vi "FTW-CodeGen-BuildMenu5.vi"(0 "State In":T2, 5 "XRef":refnum<vi>, 7 "MenuRef":refnum<k9>, 9 "Point":cluster{"H":i32, "V":i32}, 11 "Menu Type":T1(ring)) -> ()   [LabVIEW 2015, in "FTW-Dataflow-Burrow.xnode"]
uses:
  FTW-Dataflow-Burrow.xnode
  FTW-CodeGen-State.ctl
panel:
  # "Inputs"
  # "Outputs"
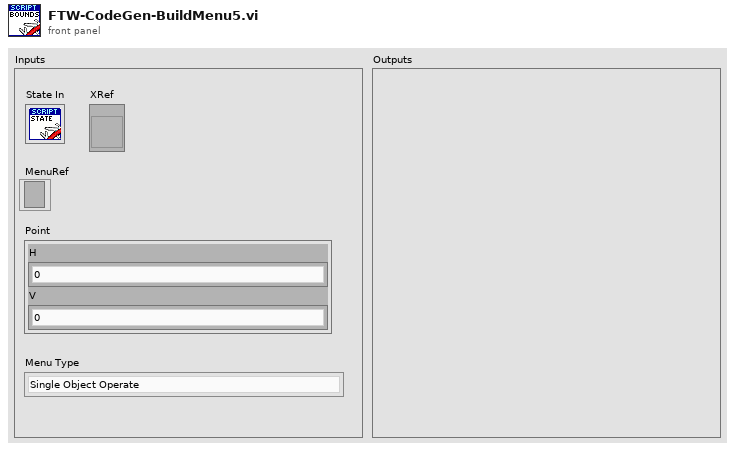
[diagram p1: front panel]
types:
  T1 = enum32{"Single Object Operate", "Single Object Popup", "Multi Object Popup Master", "Multi Object Popup Other"}
  T2 = typedef "FTW-Dataflow-Burrow.xnode/FTW-CodeGen-State.ctl" = cluster{"InputTerminals":cluster{"Wired?":bool, "ID":string, "DataName":string, "DataColor":u32, "Type":variant}[], "EnableTiming?":bool}
  T3 = cluster{"Wired?":bool, "ID":string, "DataName":string, "DataColor":u32, "Type":variant}[]
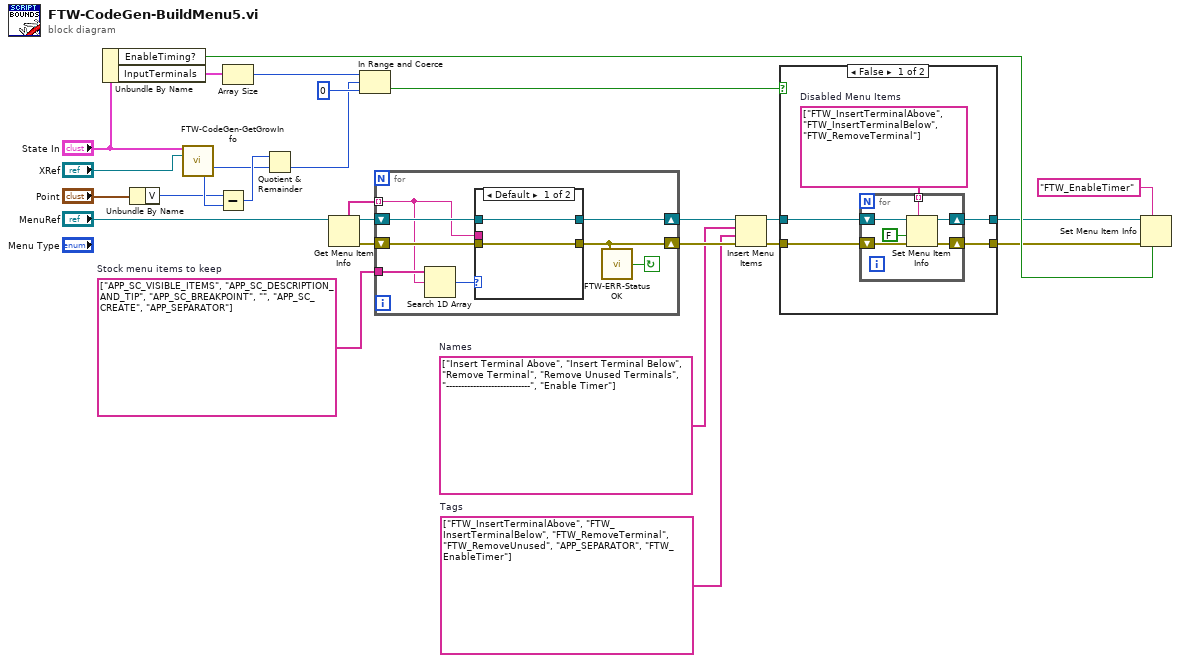
[diagram p0: block diagram]
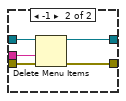
[diagram p3: hidden frame]
diagram:
  w19 = string[] ["FTW_InsertTerminalAbove", "FTW_InsertTerminalBelow", "FTW_RemoveTerminal", "FTW_RemoveUnused", "APP_SEPARATOR", "FTW_EnableTimer"]  # Tags
  w20 = string[] ["Insert Terminal Above", "Insert Terminal Below", "Remove Terminal", "Remove Unused Terminals", "----------------------------", "Enable Timer"]  # Names
  w25 = string[] ["APP_SC_VISIBLE_ITEMS", "APP_SC_DESCRIPTION_AND_TIP", "APP_SC_BREAKPOINT", "", "APP_SC_CREATE", "APP_SEPARATOR"]  # Stock menu items to keep
  n1 = Unbundle By Name("State In") -> ("EnableTiming?"=w17:bool, "InputTerminals"=w1:T3)
  n2 = Unbundle By Name("Point") -> ("V"=w13:i32)
  n3 = call "FTW-CodeGen-GetGrowInfo.vi"("State In"="State In", "XRef"="XRef") -> ("Terminal Height"=w14:i32, "Total Top Banner Height"=w16:i32)  [unwired: 5 in, 7 out]
  n4 = Subtract(x=w13, y=w16) -> (x-y=w15:i32)
  n5 = Array Size(array=w1) -> (size(s)=w8:i32)
  n6 = Quotient & Remainder(x=w15, y=w14) -> (floor(x/y)=w7:i32)  [unwired: 1 out]
  n7 = Get Menu Item Info(11:"MenuRef") -> (0:w23:errorcluster, 3:w26:refnum<k9>, 5:w24:string[])  [unwired: 2 in, 4 out]
  n8 = In Range and Coerce(upper limit=w8, x=w7, lower limit=0) -> (In Range?=w2:bool)  [unwired: 1 out]
  n9 = for {
    shift-right: [w35] -> w21
    shift-left: w26 -> [w34]
    tunnel: w25 -> [w33]
    tunnel: w24 -> [w30] mode=indexing
    shift-right: [w29] -> w22
    shift-left: w23 -> [w31]
    stop <- w28 continue-if-true
    n10 = Search 1D Array(1D array=w33, element=w30) -> (index of element=w32:i32)  [unwired: 1 in]
    n11 = case shown="Default" w32 {
      tunnel: [w37 w42] -> w35
      tunnel: w34 -> [w37 w41]
      tunnel: w31 -> [w36 w40]
      tunnel: [w36 w39] -> w29
      tunnel: w30 -> [_ w38]
      frame Default {
      }
      frame -1 {
        n12 = Delete Menu Items(6:w40, 7:w38, 9:w41) -> (0:w39:errorcluster, 3:w42:refnum<k9>)  [unwired: 1 in]
      }
    }
    n13 = call "FTW-ERR-StatusOK.vi"("error to check"=w29) -> ("Status OK?"=w28:bool)
  }
  n14 = Insert Menu Items(6:w22, 7:w19, 8:w20, 9:w21) -> (0:w5:errorcluster, 3:w6:refnum<k9>)  [unwired: 2 in, 1 out]
  n15 = case shown="False" w2 {
    tunnel: w6 -> [w47 w55]
    tunnel: w5 -> [w46 w54]
    tunnel: [w44 w55] -> w4
    tunnel: [w43 w54] -> w3
    frame False {
      w45 = string[] ["FTW_InsertTerminalAbove", "FTW_InsertTerminalBelow", "FTW_RemoveTerminal"]  # Disabled Menu Items
      n16 = for {
        shift-right: [w51] -> w44
        shift-left: w47 -> [w53]
        shift-right: [w50] -> w43
        shift-left: w46 -> [w52]
        tunnel: w45 -> [w48] mode=indexing
        n17 = Set Menu Item Info(7:w48, 8:w52, 9:FALSE ("enabled"), 11:w53) -> (0:w50:errorcluster, 3:w51:refnum<k9>)  [unwired: 3 in]
      }
    }
    frame True {
    }
  }
  n18 = Set Menu Item Info(6:w17, 7:"FTW_EnableTimer" ("item tag"), 8:w3, 11:w4) -> ()  [unwired: 3 in, 2 out]
